vi "Send to serial.vi"(8 "error in (no error)":errorcluster, 10 "message":string, 11 "Roda_Filtros in":refnum<class "Roda_Filtros.lvclass">) -> (0 "error out":errorcluster, 3 "Roda_Filtros out":refnum<class "Roda_Filtros.lvclass">)   [LabVIEW 2018, in "Roda_Filtros.lvclass"]
uses:
  Roda_Filtros.lvclass
  Roda_Filtros.lvclass/Roda_Filtros.ctl
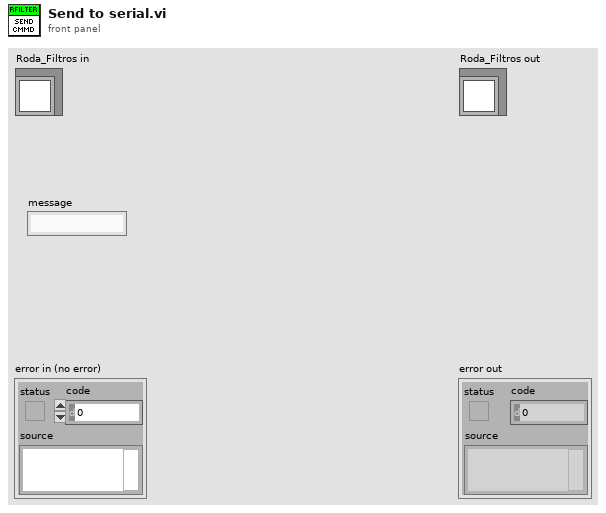
[diagram p1: front panel]
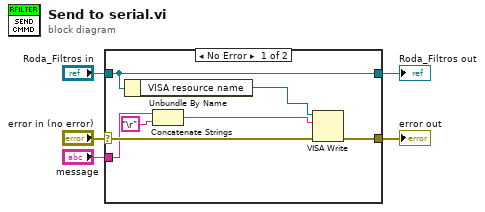
[diagram p0: block diagram]
diagram:
  n1 = case shown="No Error" "error in (no error)" {
    selector: "error in (no error)" -> [w12 w14]
    tunnel: [w11 w14] -> w4
    tunnel: [w10 w13] -> w2
    tunnel: "Roda_Filtros in" -> [w10 w13]
    tunnel: "message" -> [w8 _]
    frame No Error {
      n2 = Unbundle By Name(w10) -> ("VISA resource name"=w9:refnum<visa-resource-name>)
      n3 = Concatenate Strings(w8, "\r") -> (w6:string)
      n4 = VISA Write(VISA resource name=w9, write buffer=w6, error in (no error)=w12) -> (error out=w11:errorcluster)  [unwired: 2 out]
    }
    frame Error {
    }
  }
  "error out" <- w4
  "Roda_Filtros out" <- w2
